vi "writeDefaultValuesToDisk.vi"(1 "appFolder":path, 5 "error in (no error)":errorcluster, 7 "Control Label":string, 9 "Caption":string, 11 "Value (XML String)":string) -> (19 "error out":errorcluster)   [LabVIEW 2022 SP3, in "stillnessHelper.lvclass"]
doc: "This writes an XML file with the value using XML string as data and \"Label\" and \"Caption\" to build the file name in a given application data folder."
uses:
  stillnessHelper.lvclass
  <vilib>/Utility/xml.llb/Write to XML File(string).vi
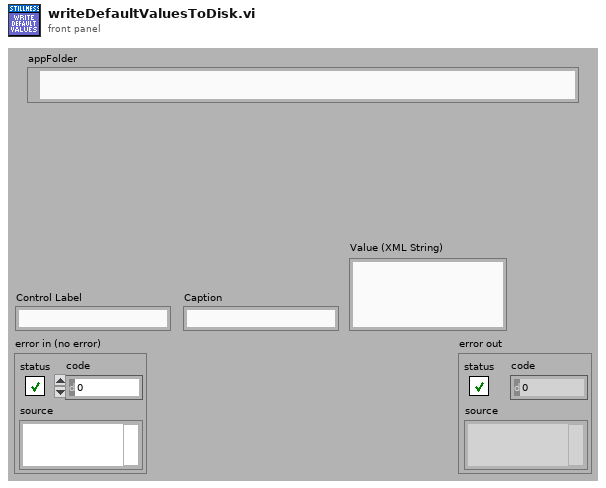
[diagram p1: front panel]
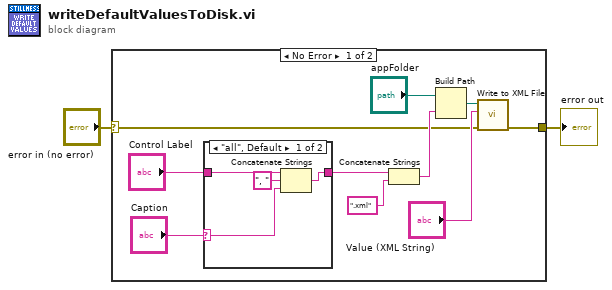
[diagram p0: block diagram]
diagram:
  n1 = case shown="No Error" "error in (no error)" {
    selector: "error in (no error)" -> [w4 w18]
    tunnel: [w5 w18] -> w1
    frame No Error {
      n2 = case shown="\"all\", Default" "Caption" {
        selector: "Caption" -> [w13 _]
        tunnel: [w16 w17] -> w7
        tunnel: "Control Label" -> [w15 w17]
        frame "all", Default {
          n3 = Concatenate Strings(w15, ", " ("string"), w13) -> (w16:string)
        }
        frame "" {
        }
      }
      n4 = Concatenate Strings(w7, ".xml" ("string")) -> (w10:string)
      n5 = Build Path(base path="appFolder", name or relative path=w10) -> (appended path=w12:path)
      n6 = call-poly <vilib>:"Write to XML File.vi"("error in (no error)"=w4, "XML Input"="Value (XML String)", "XML File Path"=w12) -> ("error out"=w5:errorcluster)  [unwired: 6 in, 2 out]
    }
    frame Error {
    }
  }
  "error out" <- w1
